vi "DAT to LV.vi"(8 "error in (no error)":errorcluster, 10 "header length":i32=11, 11 "File Path":path) -> (0 "error out":errorcluster, 2 "Data":dbl[][](array[numeric]), 3 "Data (Dictionary)":cluster{"key":variant, "value":variant}[](array[cluster]), 4 "Comments":string, 5 "Wavenames":string[](array[string]))   [LabVIEW 2016, in "LV to ITX.lvclass"]
uses:
  LV to ITX.lvclass
  <vilib>/Utility/file.llb/Read Delimited Spreadsheet (string).vi
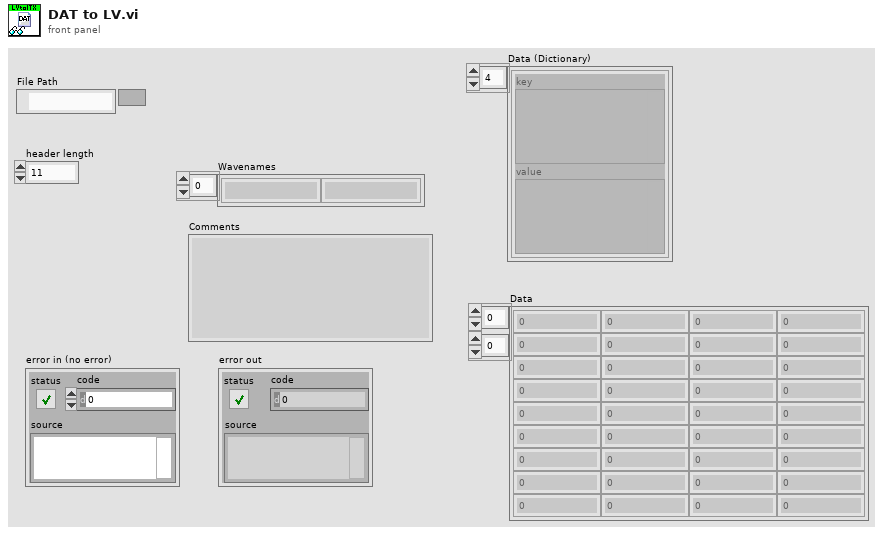
[diagram p1: front panel]
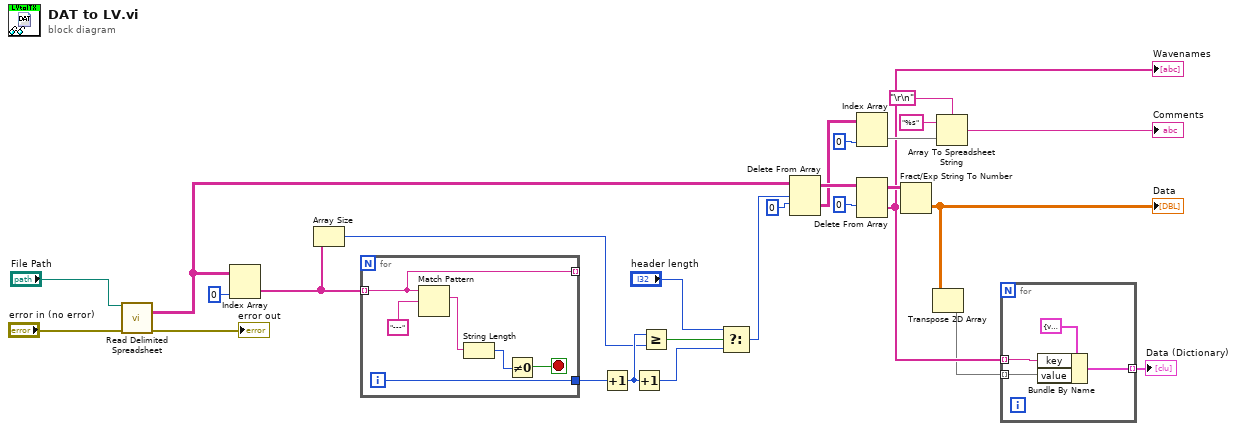
[diagram p0: block diagram]
diagram:
  n1 = call-poly <vilib>:"Read Delimited Spreadsheet.vi"("file path (dialog if empty)"="File Path", "error in (no error)"="error in (no error)") -> ("all rows"=w14:string[][], "error out"=→"error out":errorcluster)  [unwired: 8 in, 4 out]
  n2 = Index Array(array=w14, index (col)=0 ("disabled index (col)")) -> (element=w11:string[])  [unwired: 1 in]
  n3 = Array Size(array=w11) -> (size(s)=w8:i32)
  n4 = for {
    tunnel: w11 -> [w28] mode=indexing
    tunnel: [w29] -> w12
    tunnel: [w28] -> _ mode=indexing
    i -> [w29]
    stop <- w31 stop-if-true
    n5 = Match Pattern(string=w28, regular expression="---") -> (match substring=w32:string)  [unwired: 4 out]
    n6 = String Length(string=w32) -> (length=w30:i32)
    n7 = Not Equal To 0?(x=w30) -> (x != 0?=w31:bool)
  }
  n8 = Increment(x=w12) -> (x+1=w10:i32)
  n9 = Increment(x=w10) -> (x+1=w7:i32)
  n10 = Greater Or Equal?(x=w10, y=w8) -> (x >= y?=w9:bool)
  n11 = Select(t="header length", s=w9, f=w7) -> (s? t:f=w5:i32)
  n12 = Delete From Array(array=w14, length=w5, index (row)=0) -> (deleted portion=w18:string[][], array with subset deleted=w24:string[][])  [unwired: 1 in]
  n13 = Index Array(array=w18, index (col)=0 ("disabled index (col)")) -> (element=w17:string[])  [unwired: 1 in]
  n14 = Delete From Array(array=w24, index (row)=0) -> (deleted portion=w4:string[], array with subset deleted=w25:string[][])  [unwired: 2 in]
  "Wavenames" <- w4
  n15 = Fract/Exp String To Number(string=w25) -> (number=w3:dbl[][])  [unwired: 3 in, 1 out]
  "Data" <- w3
  n16 = Transpose 2D Array(2D array=w3) -> (transposed array=w1:dbl[][])
  n17 = Array To Spreadsheet String(delimiter (Tab)="\r\n", array=w17, 3:"%s" ("format string")) -> (spreadsheet string=→"Comments":string)
  n18 = for {
    tunnel: w4 -> [w36] mode=indexing
    tunnel: w1 -> [w35] mode=indexing
    tunnel: [w34] -> w2 mode=indexing
    n19 = Bundle By Name(cluster=cluster{"key":variant, "value":variant} {"key"=variant, "value"=variant} ("key-value"), "key"=w36, "value"=w35) -> (w34:cluster{"key":variant, "value":variant})
  }
  "Data (Dictionary)" <- w2
